vi "Write DAQmxTask dict.vi"(8 "error in (no error)":errorcluster, 10 "DAQmxTask dict":variant, 11 "DAQmxTaskContainer in":refnum<class "DAQmxTaskContainer.lvclass">) -> (0 "error out":errorcluster, 3 "DAQmxTaskContainer out":refnum<class "DAQmxTaskContainer.lvclass">)   [LabVIEW 2015, in "DAQmxTaskContainer.lvclass"]
uses:
  DAQmxTaskContainer.lvclass
  DAQmxTaskContainer.lvclass/DAQmxTaskContainer.ctl
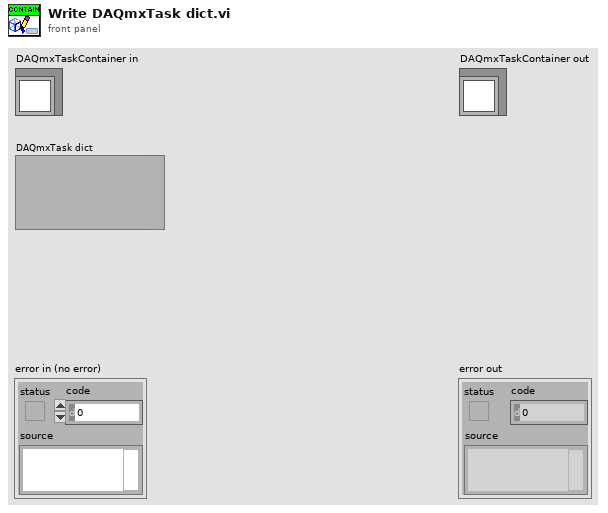
[diagram p1: front panel]
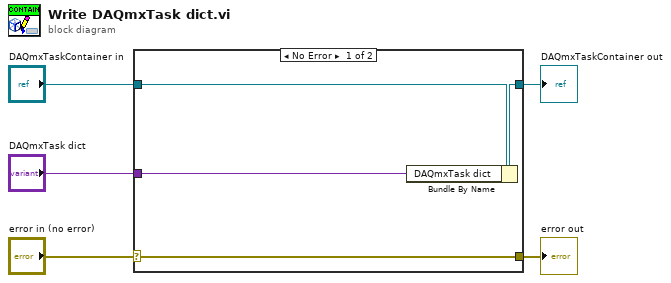
[diagram p0: block diagram]
diagram:
  n1 = case shown="No Error" "error in (no error)" {
    selector: "error in (no error)" -> [w9 w10]
    tunnel: [w9 w10] -> w4
    tunnel: [w7 w11] -> w2
    tunnel: "DAQmxTaskContainer in" -> [w8 w11]
    tunnel: "DAQmxTask dict" -> [w6 _]
    frame No Error {
      n2 = Bundle By Name(cluster=w8, "DAQmxTask dict"=w6) -> (w7:refnum<class "DAQmxTaskContainer.lvclass">)
    }
    frame Error {
    }
  }
  "error out" <- w4
  "DAQmxTaskContainer out" <- w2
